vi "FaceDetectionTester.vi"() -> ()   [LabVIEW 2017]
uses:
  Camera_IMAQdx_class/typedefs/Configuration--Cluster.ctl
  Camera_IMAQdx_class/Camera_IMAQdx.lvclass
  ImageFacialDetection_class/ImageFacialDetection.lvclass
  <userlib>/_OpenG.lib/comparison/comparison.llb/Boolean Changed__ogtk.vi
panel:
  in  "Refresh List":bool
  in  "Find Faces":bool
  in  "Connect to Camera":bool
  in  "Cameras":u16(ring) items=["VMware Virtual USB Video Device "]
  out "Image":picture
  in  "OK":bool
  out "Frame Number:":u32
  out "Connected":bool
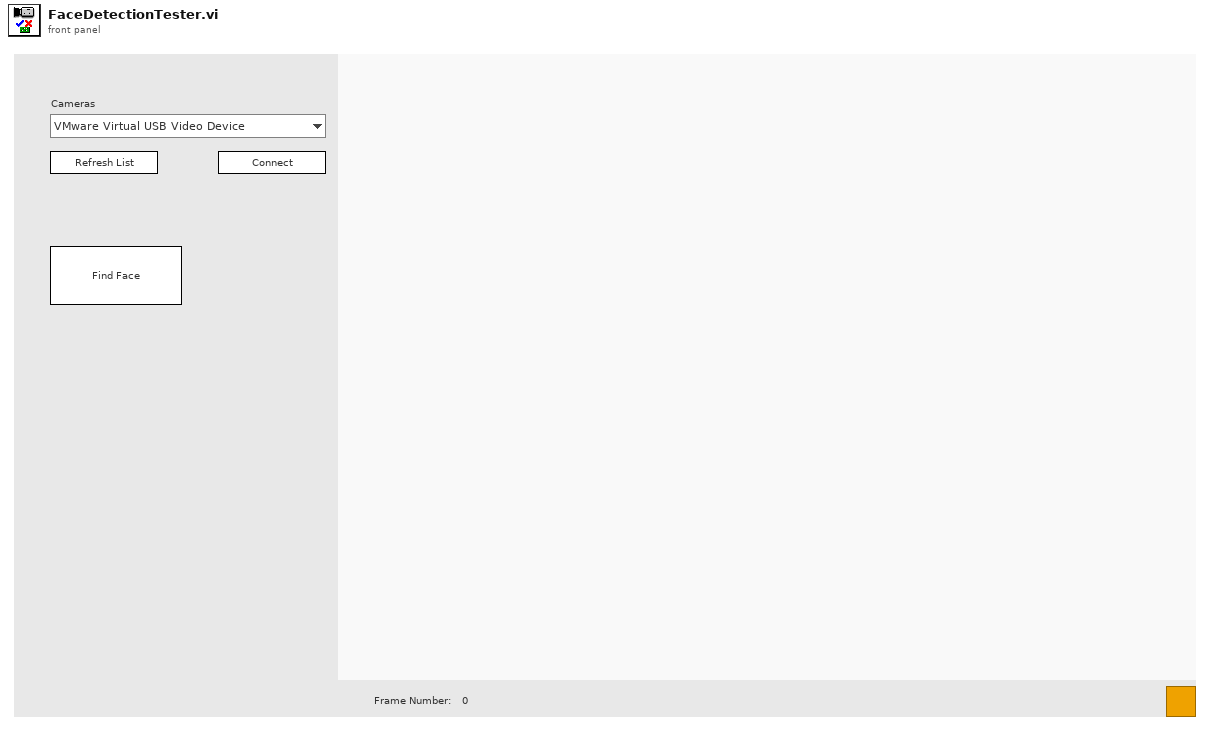
[diagram p1: front panel]
types:
  T1 = typedef "Camera_IMAQdx.lvclass/Configuration--Cluster.ctl" = cluster{"Camera Interface Name":string, "Number of Buffers":u32, "Image Name":string}
  T2 = enum32{"invalid app kind", "Development System", "Run Time System", "Student Edition", "Embedded LabVIEW", "Evaluation", "Custom"}
  T3 = enum8{"Enabled", "Disabled", "Disabled and Grayed Out"}
  T4 = enum32{"Invalid", "Standard", "Closed", "Hidden", "Minimized", "Maximized"}
  T5 = cluster{"Core":cluster{"Current VI Reference":refnum<vi>, "Close Panel on Exit?":bool}, "Camera.IMAQdx":refnum<class "Camera_IMAQdx.lvclass">, "All Camera Interfaces":string[], "Connected":bool, "Grabbing":bool, "ImageFacialDetection":refnum<class "ImageFacialDetection.lvclass">}
  T6 = cluster{"Current VI Reference":refnum<vi>, "Close Panel on Exit?":bool}
  T7 = typedef "IMAQ Image.ctl" = refnum<image>
  T8 = cluster{"Type":u32, "Version":u32, "Flags":u32, "SerialNumberHigh":u32, "SerialNumberLow":u32, "BusType":u32, "InterfaceName":string, "VendorName":string, "ModelName":string, "CameraFileName":string, "CameraAttributeURL":string}[]
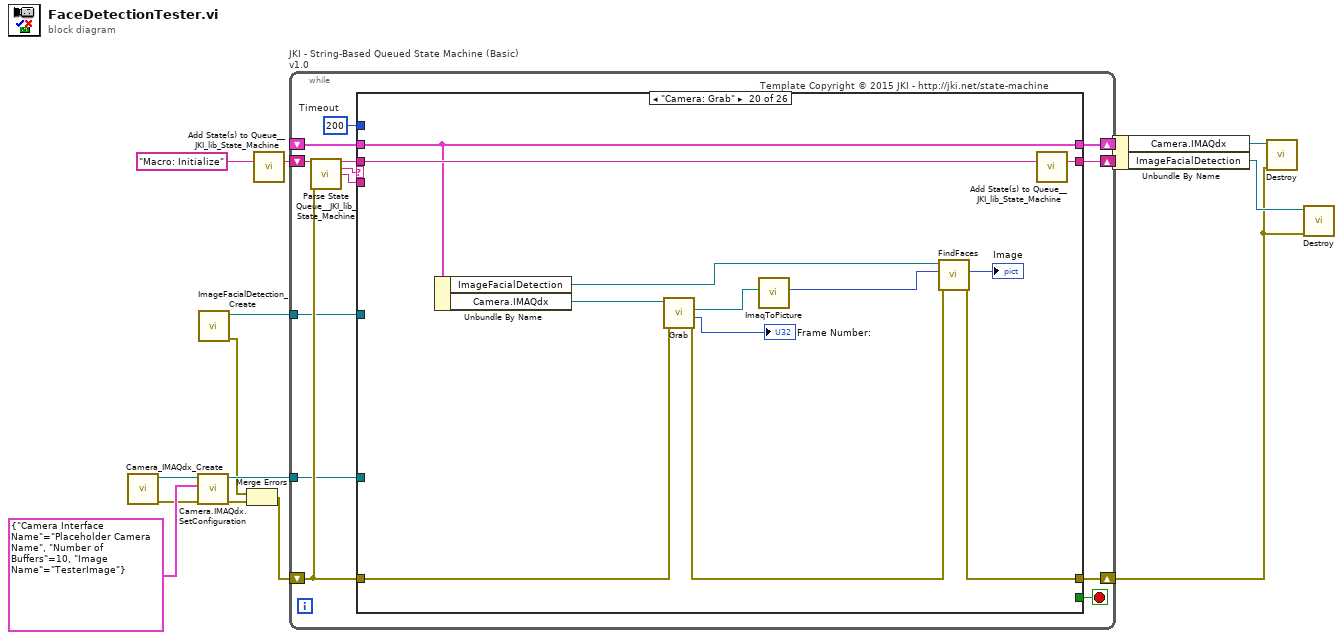
[diagram p0: block diagram]
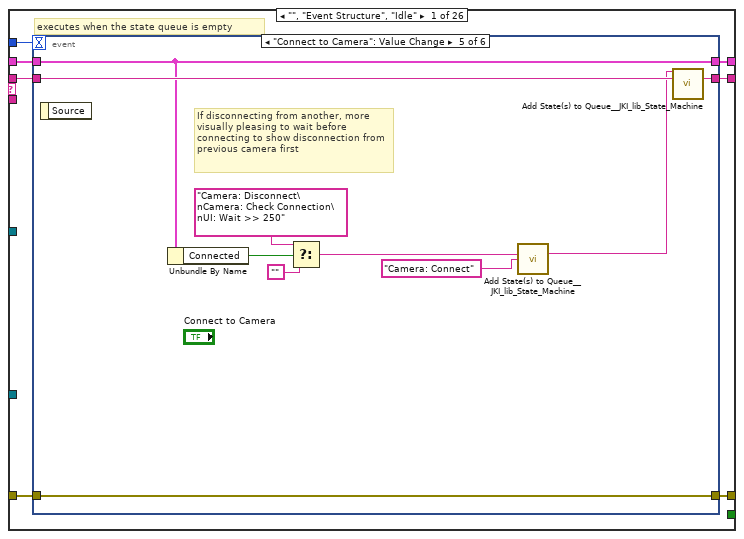
[diagram p2: hidden frame]
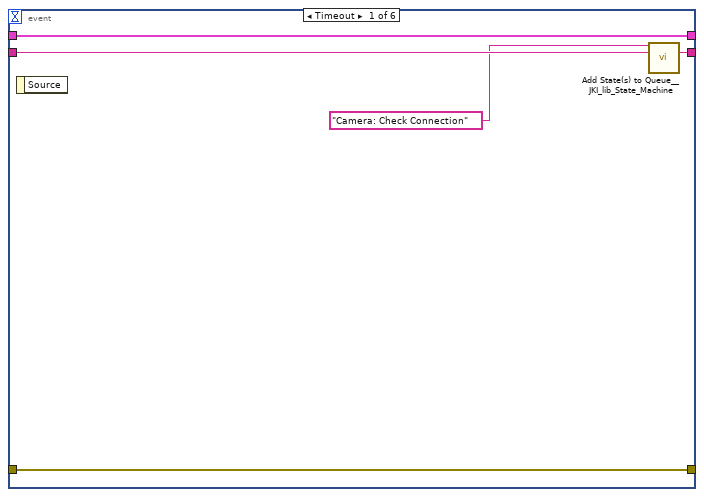
[diagram p3: hidden frame]
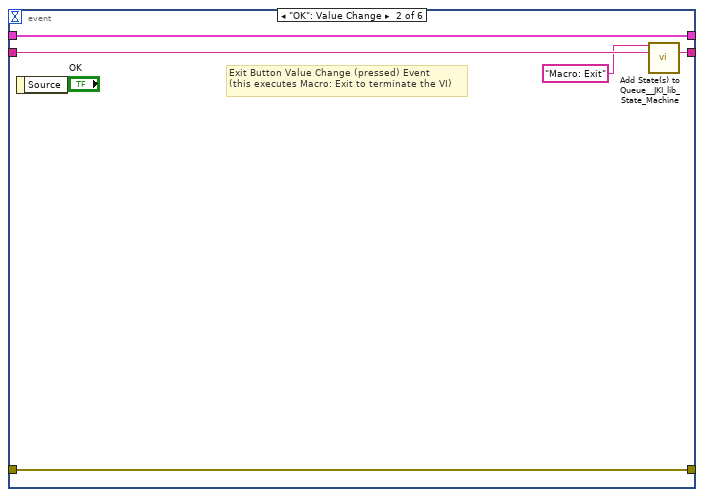
[diagram p4: hidden frame]
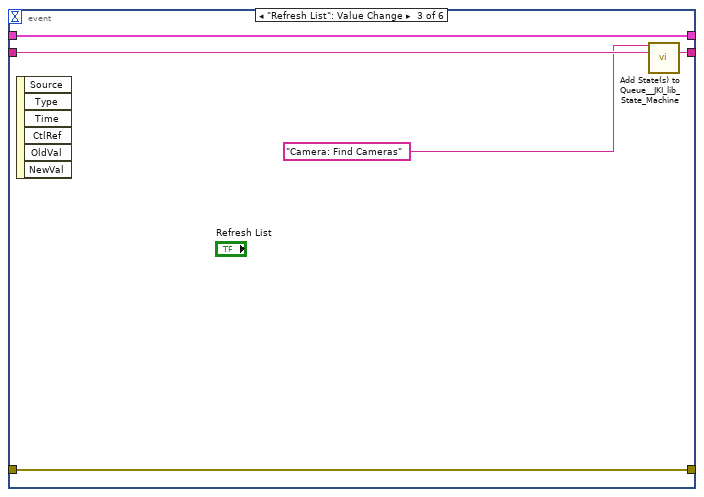
[diagram p5: hidden frame]
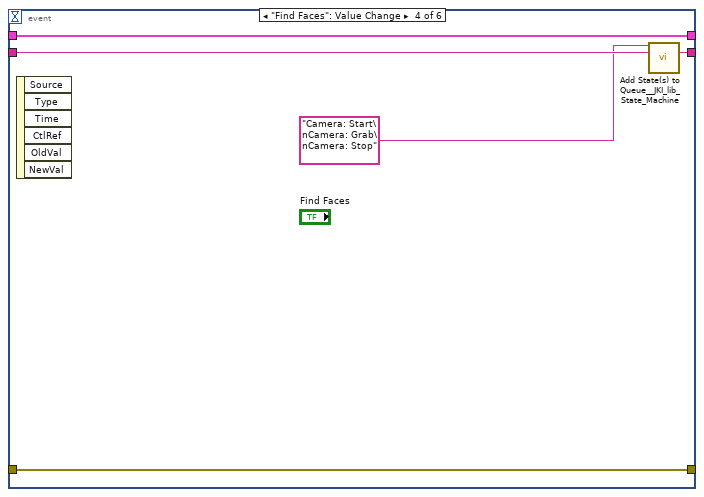
[diagram p6: hidden frame]
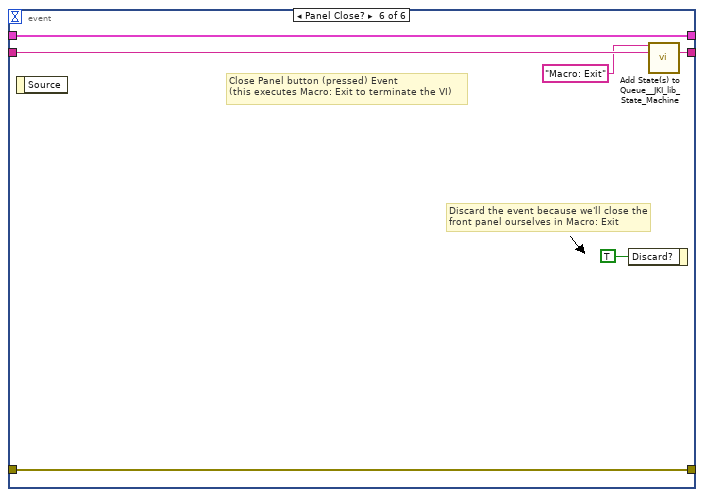
[diagram p7: hidden frame]
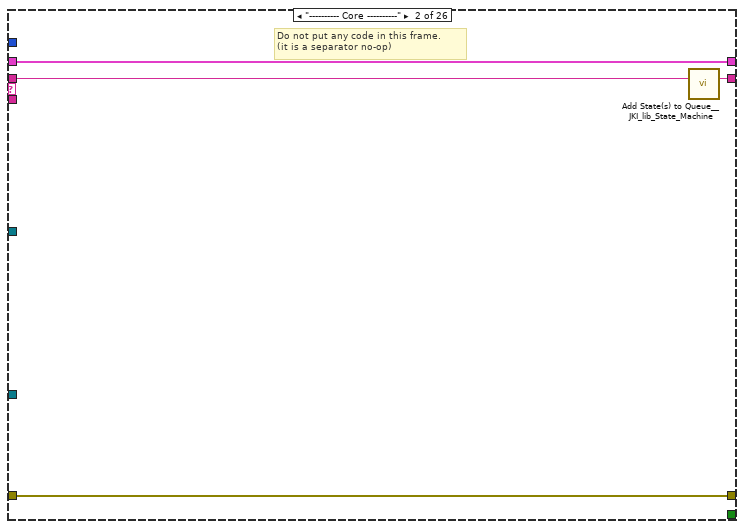
[diagram p8: hidden frame]
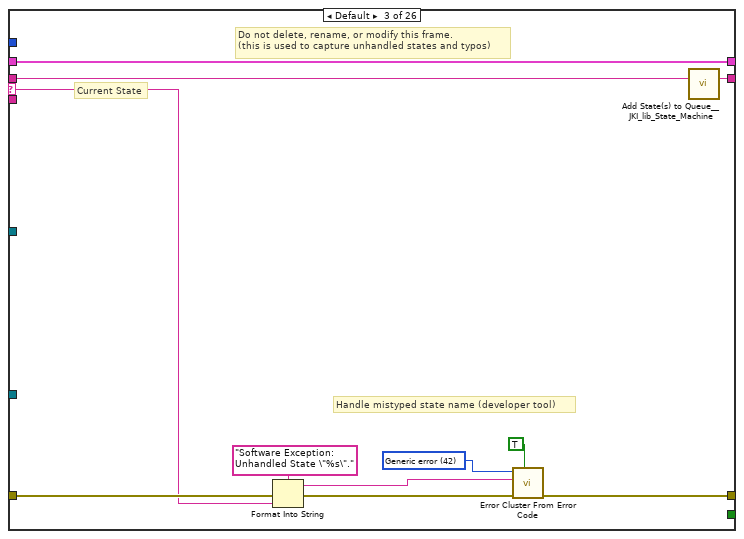
[diagram p9: hidden frame]
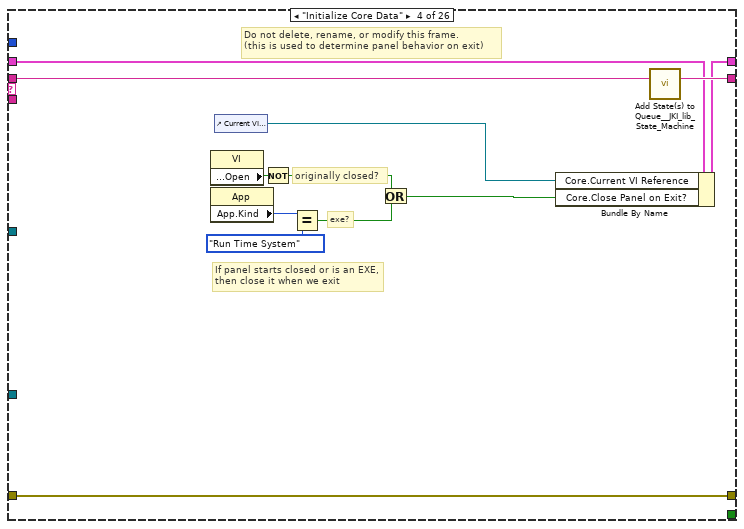
[diagram p10: hidden frame]
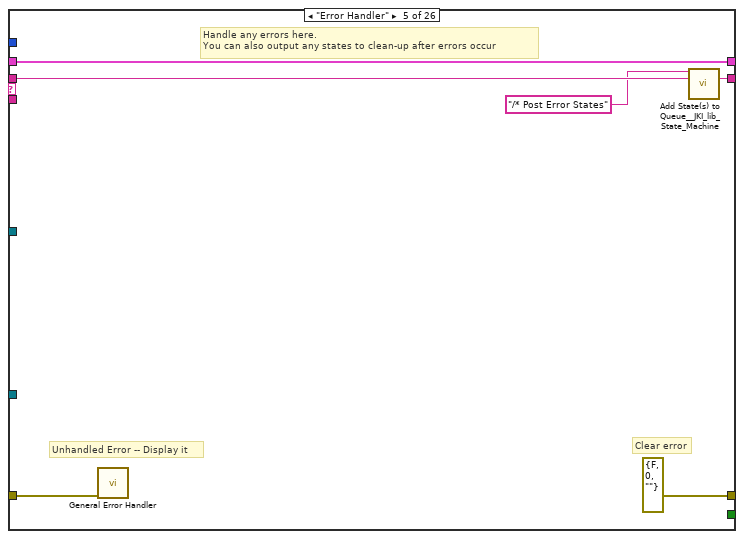
[diagram p11: hidden frame]
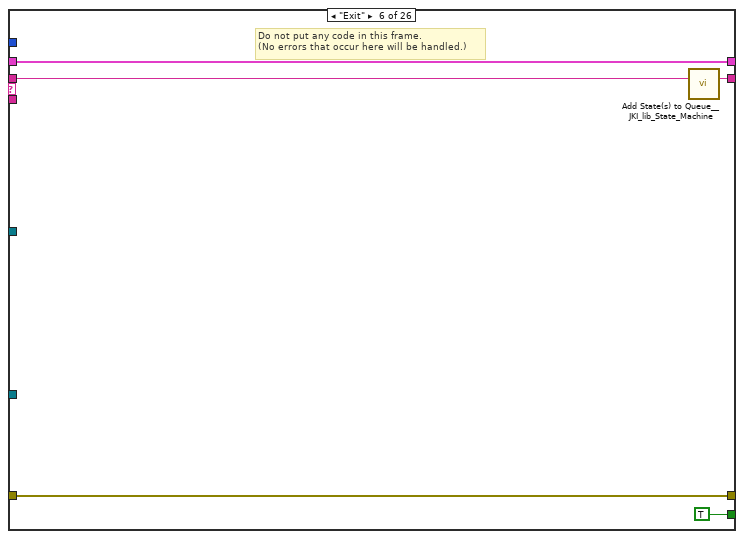
[diagram p12: hidden frame]
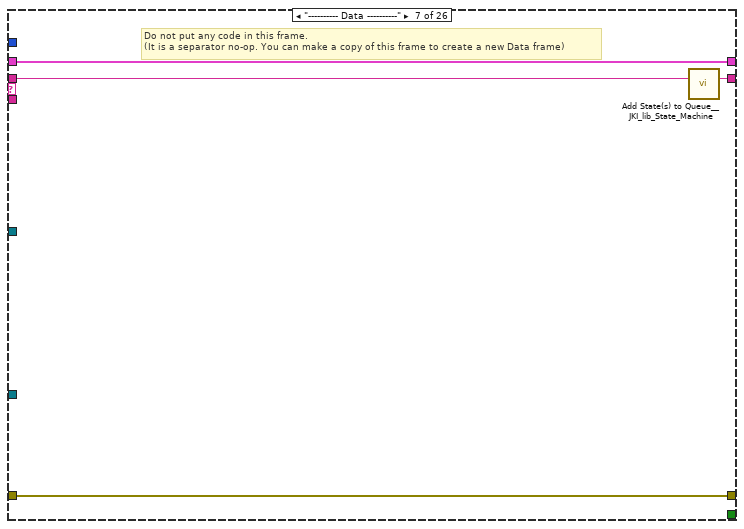
[diagram p13: hidden frame]
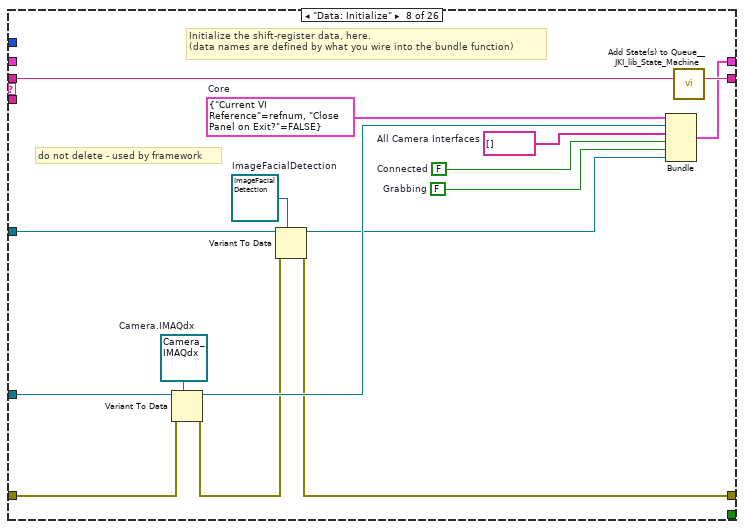
[diagram p14: hidden frame]
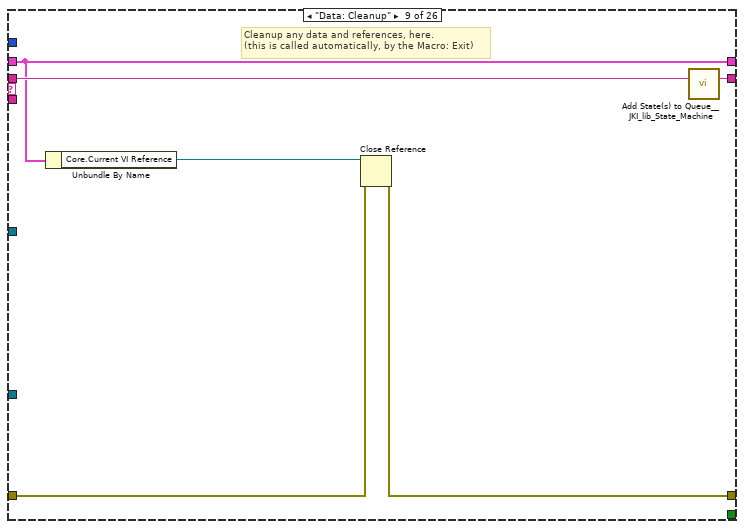
[diagram p15: hidden frame]
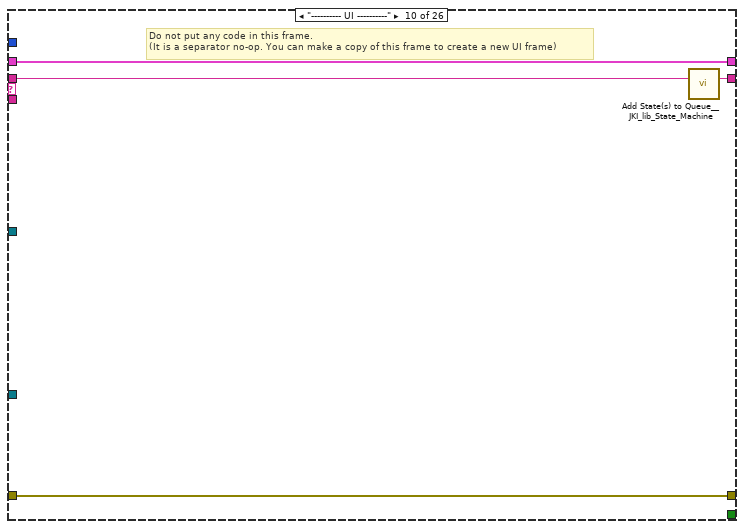
[diagram p16: hidden frame]
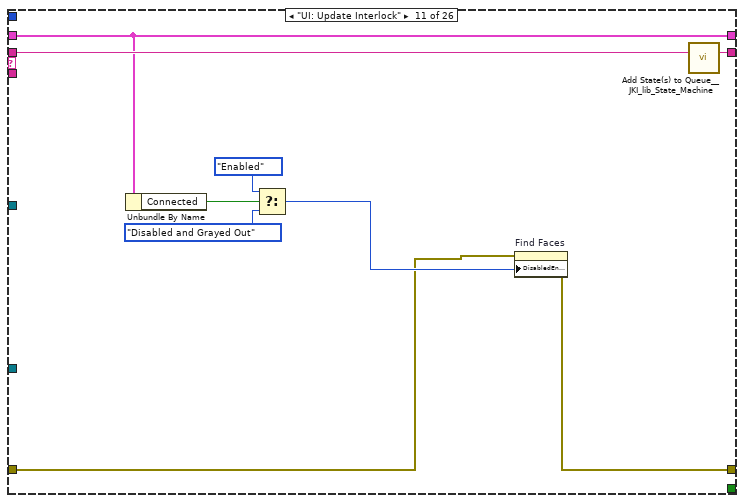
[diagram p17: hidden frame]
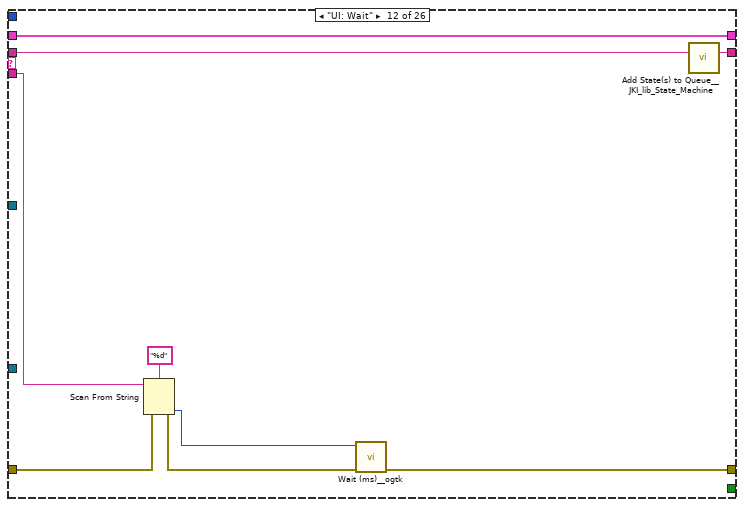
[diagram p18: hidden frame]
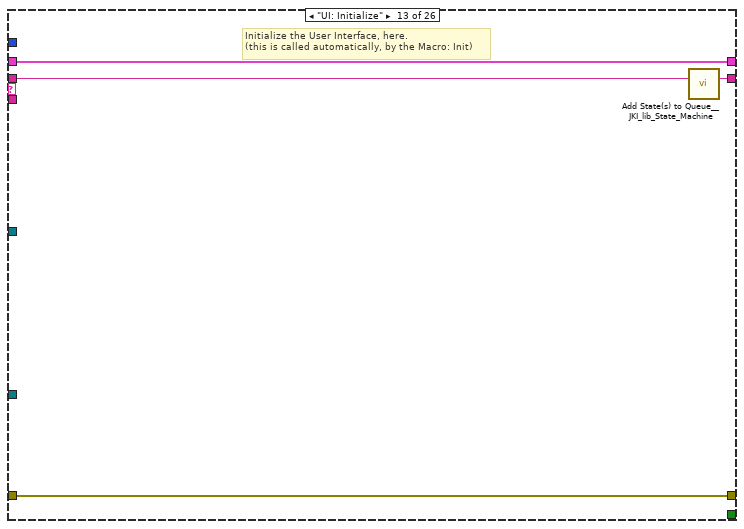
[diagram p19: hidden frame]
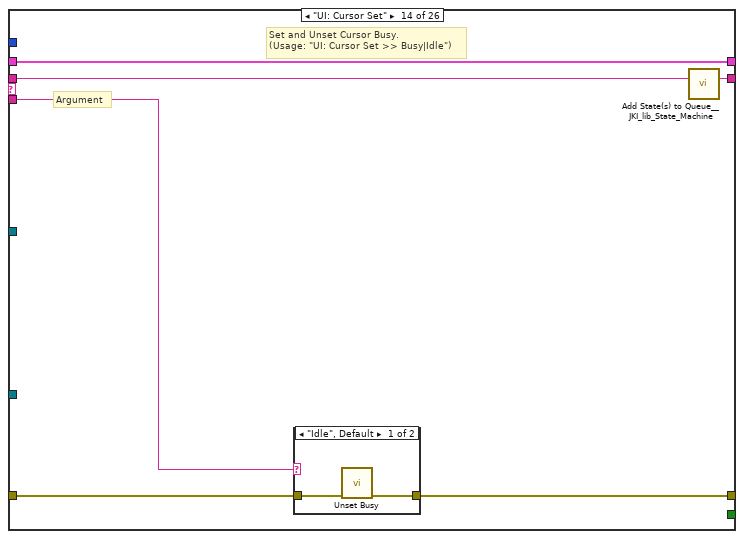
[diagram p20: hidden frame]
diagram:
  n1 = call "Camera_IMAQdx_Create.vi"() -> ("error out"=w7:errorcluster, "reference out"=w12:refnum<class "Camera_IMAQdx.lvclass">)  [unwired: 10 in]
  n2 = call "Camera.IMAQdx.SetConfiguration.vi"("error in (no error)"=w7, "Configuration"=T1 {"Camera Interface Name"="Placeholder Camera Name", "Number of Buffers"=10, "Image Name"="TesterImage"}, "reference in"=w12) -> ("error out"=w6:errorcluster, "reference out"=w9:refnum<class "Camera_IMAQdx.lvclass">)  [unwired: 7 in]
  n3 = call "ImageFacialDetection_Create.vi"() -> ("error out"=w3:errorcluster, "reference out"=w5:refnum<class "ImageFacialDetection.lvclass">)  [unwired: 10 in]
  n4 = Merge Errors(w3, w6) -> (w4:errorcluster)
  n5 = call <vilib>:"Add State(s) to Queue__JKI_lib_State_Machine.vi"("State(s) in (\"\")"="Macro: Initialize") -> ("States Out"=w14:string)  [unwired: 14 in]
  n6 = while "JKI - String-Based Queued State Machine (Basic) v1.0" {
    shift-right: [w20] -> w11
    shift-left: _ -> [w19]
    shift-right: [w23] -> w1
    shift-left: w4 -> [w17]
    shift-right: [w22] -> _
    shift-left: w14 -> [w24]
    tunnel: w9 -> [w16]
    tunnel: w5 -> [w15]
    stop <- w21 stop-if-true
    w18 = 200  # Timeout
    # "Template Copyright © 2015 JKI - http://jki.net/state-machine"
    n7 = call <vilib>:"Parse State Queue__JKI_lib_State_Machine.vi"("State Queue"=w24, "Error In (no error)"=w17) -> ("Remaining States"=w26:string, "Current State"=w27:string, "Arguments"=w25:string)  [unwired: 11 in]
    n8 = case shown="\"Camera: Grab\"" w27 {
      selector: w27 -> [_ _ w75 _ _ _ _ _ _ _ _ _ _ _ _ _ _ _ _ _ _ _ _ _ _ _]
      tunnel: w26 -> [w34 w74 w79 w97 w103 w108 w112 w128 w134 w138 w147 w156 w160 w166 w177 w203 w208 w227 w231 w243 w255 w264 w273 w284 w301 w307]
      tunnel: w25 -> [_ _ _ _ _ _ _ _ _ _ _ w152 _ w161 w171 _ _ _ _ _ _ _ _ _ _ _]
      tunnel: w19 -> [w32 w71 w77 w88 w100 w106 w109 _ w129 w135 w145 w154 w158 w164 w173 w200 w205 w224 w228 w241 w250 w257 w268 w276 w299 w305]
      tunnel: [w31 w72 w81 w94 errorcluster {"status"=FALSE, "code"=0, "source"=""} ("error out") w105 w110 w113 w130 w136 w140 w153 w157 w162 w174 w201 w206 w225 w229 w232 w251 w260 w269 w279 w291 w302] -> w23
      tunnel: w17 -> [w30 w72 w80 w94 w99 w105 w110 w120 w131 w136 w139 w149 w157 w163 w175 w201 w206 w225 w229 w239 w252 w261 w270 w278 w293 w303]
      tunnel: [w33 w73 w78 w96 w102 w107 w111 w127 w133 w137 w146 w155 w159 w165 w176 w202 w207 w226 w230 w242 w254 w263 w272 w283 w300 w306] -> w22
      tunnel: [_ _ _ _ _ TRUE _ _ _ _ _ _ _ _ _ _ _ _ _ _ _ _ _ _ _ _] -> w21
      tunnel: [w29 w71 w77 w95 w100 w106 w109 w126 w129 w135 w145 w154 w158 w164 w173 w200 w205 w224 w228 w241 w249 w256 w267 w275 w299 w305] -> w20
      tunnel: w18 -> [w28 _ _ _ _ _ _ _ _ _ _ _ _ _ _ _ _ _ _ _ _ _ _ _ _ _]
      tunnel: w16 -> [_ _ _ _ _ _ _ w124 _ _ _ _ _ _ _ _ _ _ _ _ _ _ _ _ _ _]
      tunnel: w15 -> [_ _ _ _ _ _ _ w116 _ _ _ _ _ _ _ _ _ _ _ _ _ _ _ _ _ _]
      frame "", "Event Structure", "Idle" {
        # "executes when the state queue is empty"
        n9 = event shown="[4] \"Connect to Camera\": Value Change" {
          selector: _ -> [_ _ _ _ _ _]
          dyn-events: _ -> [_ _ _ _ _ _]
          timeout: w28 -> [_ _ _ _ _ _]
          tunnel: w34 -> [w39 w44 w49 w54 w64 w70]
          tunnel: [w38 w43 w48 w53 w63 w69] -> w33
          tunnel: w32 -> [w36 w41 w46 w51 w61 w67]
          tunnel: [w37 w42 w47 w52 w62 w68] -> w31
          tunnel: w30 -> [w37 w42 w47 w52 w62 w68]
          tunnel: [w36 w41 w46 w51 w61 w67] -> w29
          event Timeout {
            n10 = event-data() -> ()  [unwired: 1 in, 1 out]
            n11 = call <vilib>:"Add State(s) to Queue__JKI_lib_State_Machine.vi"("State(s) in Front (\"\")"="Camera: Check Connection", "State(s) in (\"\")"=w39) -> ("States Out"=w38:string)  [unwired: 13 in]
          }
          event "OK": Value Change {
            # "Exit Button Value Change (pressed) Event\n(this executes Macro: Exit to terminate the VI)"
            n12 = event-data() -> ()  [unwired: 1 in, 1 out]
            n13 = call <vilib>:"Add State(s) to Queue__JKI_lib_State_Machine.vi"("State(s) in Front (\"\")"="Macro: Exit", "State(s) in (\"\")"=w44) -> ("States Out"=w43:string)  [unwired: 13 in]
          }
          event "Refresh List": Value Change {
            n14 = event-data() -> ()  [unwired: 1 in, 6 out]
            n15 = call <vilib>:"Add State(s) to Queue__JKI_lib_State_Machine.vi"("State(s) in Front (\"\")"="Camera: Find Cameras", "State(s) in (\"\")"=w49) -> ("States Out"=w48:string)  [unwired: 13 in]
          }
          event "Find Faces": Value Change {
            n16 = event-data() -> ()  [unwired: 1 in, 6 out]
            n17 = call <vilib>:"Add State(s) to Queue__JKI_lib_State_Machine.vi"("State(s) in Front (\"\")"="Camera: Start\nCamera: Grab\nCamera: Stop", "State(s) in (\"\")"=w54) -> ("States Out"=w53:string)  [unwired: 13 in]
          }
          event "Connect to Camera": Value Change {
            # "If disconnecting from another, more visually pleasing to wait before connecting to show disconnection from previous camera first"
            n18 = event-data() -> ()  [unwired: 1 in, 1 out]
            n19 = Unbundle By Name(w61) -> ("Connected"=w60:bool)
            n20 = Select(t="Camera: Disconnect\nCamera: Check Connection\nUI: Wait >> 250", s=w60, f="") -> (s? t:f=w57:string)
            n21 = call <vilib>:"Add State(s) to Queue__JKI_lib_State_Machine.vi"("State(s) in (\"\")"=w57, "State(s) at Back (\"\")"="Camera: Connect") -> ("States Out"=w55:string)  [unwired: 13 in]
            n22 = call <vilib>:"Add State(s) to Queue__JKI_lib_State_Machine.vi"("State(s) in Front (\"\")"=w55, "State(s) in (\"\")"=w64) -> ("States Out"=w63:string)  [unwired: 13 in]
          }
          event Panel Close? {
            # "Discard the event because we'll close the front panel ourselves in Macro: Exit"
            # "Close Panel button (pressed) Event\n(this executes Macro: Exit to terminate the VI)"
            n23 = event-data() -> ()  [unwired: 1 in, 1 out]
            n24 = event-data("Discard?"=TRUE) -> ()  [unwired: 1 in, 1 out]
            n25 = call <vilib>:"Add State(s) to Queue__JKI_lib_State_Machine.vi"("State(s) in Front (\"\")"="Macro: Exit", "State(s) in (\"\")"=w70) -> ("States Out"=w69:string)  [unwired: 13 in]
          }
        }
      }
      frame "---------- Core ----------" {
        # "Do not put any code in this frame.\n(it is a separator no-op)"
        n26 = call <vilib>:"Add State(s) to Queue__JKI_lib_State_Machine.vi"("State(s) in (\"\")"=w74) -> ("States Out"=w73:string)  [unwired: 14 in]
      }
      frame Default {
        w84 = 42 items=["No error", "Argument error", "Memory is full", "Out of zone", "End of file", "File already open", "Generic file I/O error", "File not found", "File permission error", "Disk is full", "Duplicate path", "Too many files open", "System feature not enabled", "Resource file not found", "Cannot add resource", "Resource not found", "Image not found", "Image memory error", "Pen does not exist", "Config type invalid", "Config token not found", "Config parse error", "Config memory error", "Bad external code format", "Bad external code offset", "External code not present", "Null window", "Destroy window error", "Null menu", "Print aborted", "Bad print record", "Print driver error", "Windows error during printing", "Memory error during printing", "Print dialog error", "Generic print error", "Invalid device refnum", "Device not found", "Device parameter error", "Device unit error", "Cannot open device", "Device call aborted", "Generic error", "Cancelled by user", "Object ID too low", "Object ID too high", "Object not in heap", "Unknown heap", "Unknown object (invalid DefProc)", "Unknown object (DefProc not in table)", "Message out of range", "Invalid (null) method", "Unknown message", "Manager call not supported", "Bad address", "Network operation in progress", "Network operation timed out", "Connection is busy", "Network attribute not supported", "Network error", "Address in use", "System out of memory", "Connection aborted", "Connection refused", "Not connected", "Already connected", "Connection closed", "Initialization error (interapplication manager)", "Bad occurrence", "Wait on unbound occurrence handler", "Occurrence queue overflow", "Datalog type conflict", "Unused", "Unrecognized type (interapplication manager)", "Memory corrupt", "Failed to make temporary DLL", "Old CIN version", "Drag socket not found", "Failed to load drop-object", "Failed to register OLE object", "Failed to release OLE object", "Format specifier type mismatch", "Unknown format specifier", "Too few format specifiers", "Too many format specifiers", "Scan failed", "Newer CIN version", "Error converting to variant", "Runtime menu error", "Password tampered", "Variant attribute not found", "Incompatible variant data type", "Event data is not available", "Event Store is not present", "Occurrence is not found", "Event Queue is not created", "Event info is not available", "Refnum passed is NULL", "Error retrieving Class GUID", "Error retrieving CoClass GUID", "Error retrieving TypeLib GUID.", "Bad built application magic bytes.", "Specific driver is different from the specific driver associated with the Logical Name.", "There is no session opened to the class driver.", "Max Error", "MAX - Error with config objects", "MAX - Error loading configuration", "MAX - Group not supported"]
        # "Current State"
        # "Do not delete, rename, or modify this frame.\n(this is used to capture unhandled states and typos)"
        # "Handle mistyped state name (developer tool)"
        n27 = Format Into String(format string="Software Exception: Unhandled State \"%s\"." ("message"), error in=w80, w75) -> (resulting string=w83:string, error out=w82:errorcluster)  [unwired: 1 in]
        n28 = call <vilib>:"Error Cluster From Error Code.vi"("show call chain? (False)"=TRUE, "error in (no error)"=w82, "error message (\"\")"=w83, "error code (0)"=w84) -> ("error out"=w81:errorcluster)  [unwired: 5 in]
        n29 = call <vilib>:"Add State(s) to Queue__JKI_lib_State_Machine.vi"("State(s) in (\"\")"=w79) -> ("States Out"=w78:string)  [unwired: 14 in]
      }
      frame "Initialize Core Data" {
        # "Do not delete, rename, or modify this frame.\n(this is used to determine panel behavior on exit)"
        # "originally closed?"
        # "exe?"
        # "If panel starts closed or is an EXE, then close it when we exit"
        n30 = property class="VI"() -> ("Front Panel.Open"=w93:bool)  [unwired: 2 in, 2 out]
        n31 = property class="App"() -> ("App.Kind"=w92:T2)  [unwired: 2 in, 2 out]
        n32 = control-ref of="Current VI Reference"() -> (w86:refnum<vi>)
        n33 = Not(x=w93) -> (.not. x?=w90:bool)
        n34 = Equal?(x=w92, y=T2."Run Time System" ("Application:Kind")) -> (x = y?=w89:bool)
        n35 = Or(x=w90, y=w89) -> (x .or. y?=w87:bool)
        n36 = Bundle By Name(cluster=w88, "Core.Current VI Reference"=w86, "Core.Close Panel on Exit?"=w87) -> (w95:T5)
        n37 = call <vilib>:"Add State(s) to Queue__JKI_lib_State_Machine.vi"("State(s) in (\"\")"=w97) -> ("States Out"=w96:string)  [unwired: 14 in]
      }
      frame "Error Handler" {
        # "Unhandled Error -- Display it"
        # "Handle any errors here.\nYou can also output any states to clean-up after errors occur"
        # "Clear error"
        n38 = call <vilib>:"General Error Handler.vi"("error in (no error)"=w99) -> ()  [unwired: 10 in, 5 out]
        n39 = call <vilib>:"Add State(s) to Queue__JKI_lib_State_Machine.vi"("State(s) in Front (\"\")"="/* Post Error States", "State(s) in (\"\")"=w103) -> ("States Out"=w102:string)  [unwired: 13 in]
      }
      frame "Exit" {
        # "Do not put any code in this frame.\n(No errors that occur here will be handled.)"
        n40 = call <vilib>:"Add State(s) to Queue__JKI_lib_State_Machine.vi"("State(s) in (\"\")"=w108) -> ("States Out"=w107:string)  [unwired: 14 in]
      }
      frame "---------- Data ----------" {
        # "Do not put any code in this frame.\n(It is a separator no-op. You can make a copy of this frame to create a new Data frame)"
        n41 = call <vilib>:"Add State(s) to Queue__JKI_lib_State_Machine.vi"("State(s) in (\"\")"=w112) -> ("States Out"=w111:string)  [unwired: 14 in]
      }
      frame "Data: Initialize" {
        w117 = refnum<class "ImageFacialDetection.lvclass"> refnum  # ImageFacialDetection
        w118 = FALSE  # Grabbing
        w119 = FALSE  # Connected
        w122 = refnum<class "Camera_IMAQdx.lvclass"> refnum  # Camera.IMAQdx
        w123 = string[] []  # All Camera Interfaces
        w125 = T6 {"Current VI Reference"=refnum, "Close Panel on Exit?"=FALSE}  # Core
        # "do not delete - used by framework"
        # "Initialize the shift-register data, here.\n(data names are defined by what you wire into the bundle function)"
        n42 = Variant To Data(error in=w120, type=w122, Variant=w124) -> (data=w121:refnum<class "Camera_IMAQdx.lvclass">, error out=w114:errorcluster)
        n43 = Variant To Data(error in=w114, type=w117, Variant=w116) -> (data=w115:refnum<class "ImageFacialDetection.lvclass">, error out=w113:errorcluster)
        n44 = Bundle("Core"=w125, "Camera.IMAQdx"=w121, "All Camera Interfaces"=w123, "Connected"=w119, "Grabbing"=w118, "ImageFacialDetection"=w115) -> (w126:T5)  [unwired: 1 in]
        n45 = call <vilib>:"Add State(s) to Queue__JKI_lib_State_Machine.vi"("State(s) in (\"\")"=w128) -> ("States Out"=w127:string)  [unwired: 14 in]
      }
      frame "Data: Cleanup" {
        # "Cleanup any data and references, here.\n(this is called automatically, by the Macro: Exit)"
        n46 = Unbundle By Name(w129) -> ("Core.Current VI Reference"=w132:refnum<vi>)
        n47 = Close Reference(reference=w132, error in (no error)=w131) -> (error out=w130:errorcluster)
        n48 = call <vilib>:"Add State(s) to Queue__JKI_lib_State_Machine.vi"("State(s) in (\"\")"=w134) -> ("States Out"=w133:string)  [unwired: 14 in]
      }
      frame "---------- UI ----------" {
        # "Do not put any code in this frame.\n(It is a separator no-op. You can make a copy of this frame to create a new UI frame)"
        n49 = call <vilib>:"Add State(s) to Queue__JKI_lib_State_Machine.vi"("State(s) in (\"\")"=w138) -> ("States Out"=w137:string)  [unwired: 14 in]
      }
      frame "UI: Update Interlock" {
        n50 = Unbundle By Name(w145) -> ("Connected"=w144:bool)
        n51 = Select(t=T3."Enabled" ("Disabled"), s=w144, f=T3."Disabled and Grayed Out" ("Disabled")) -> (s? t:f=w141:T3)
        n52 = property on="Find Faces" class="Bool"(error in=w139, "DisabledEnum"=w141) -> (error out=w140:errorcluster)  [unwired: 1 in, 1 out]
        n53 = call <vilib>:"Add State(s) to Queue__JKI_lib_State_Machine.vi"("State(s) in (\"\")"=w147) -> ("States Out"=w146:string)  [unwired: 14 in]
      }
      frame "UI: Wait" {
        n54 = Scan From String(format string="%d", input string=w152, error in=w149) -> (error out=w148:errorcluster, output 1=w150:i32)  [unwired: 2 in, 2 out]
        n55 = call <userlib>:"Wait (ms)__ogtk.vi"("error in (no error)"=w148, "milliseconds to wait"=w150) -> ("error out"=w153:errorcluster)  [unwired: 8 in, 1 out]
        n56 = call <vilib>:"Add State(s) to Queue__JKI_lib_State_Machine.vi"("State(s) in (\"\")"=w156) -> ("States Out"=w155:string)  [unwired: 14 in]
      }
      frame "UI: Initialize" {
        # "Initialize the User Interface, here.\n(this is called automatically, by the Macro: Init)"
        n57 = call <vilib>:"Add State(s) to Queue__JKI_lib_State_Machine.vi"("State(s) in (\"\")"=w160) -> ("States Out"=w159:string)  [unwired: 14 in]
      }
      frame "UI: Cursor Set" {
        # "Argument"
        # "Set and Unset Cursor Busy.\n(Usage: \"UI: Cursor Set >> Busy|Idle\")"
        n58 = case shown="\"Idle\", Default" w161 {
          tunnel: w163 -> [w168 w170]
          tunnel: [w167 w169] -> w162
          frame "Idle", Default {
            n59 = call <vilib>:"Unset Busy.vi"("error in (no error)"=w168) -> ("error out"=w167:errorcluster)  [unwired: 10 in]
          }
          frame "Busy" {
            n60 = call <vilib>:"Set Busy.vi"("error in (no error)"=w170) -> ("error out"=w169:errorcluster)  [unwired: 9 in, 1 out]
          }
        }
        n61 = call <vilib>:"Add State(s) to Queue__JKI_lib_State_Machine.vi"("State(s) in (\"\")"=w166) -> ("States Out"=w165:string)  [unwired: 14 in]
      }
      frame "UI: Front Panel State" {
        # "Argument"
        # "Set Front Panel Open or Closed\n(Usage: \"UI: Front Panel State >> Open|Close\")"
        n62 = Unbundle By Name(w173) -> ("Core.Current VI Reference"=w172:refnum<vi>)
        n63 = case shown="\"Open\", Default" w171 {
          tunnel: w175 -> [w181 w194]
          tunnel: [w183 w195] -> w174
          tunnel: w172 -> [w182 w192]
          frame "Open", Default {
            n64 = property class="VI"(reference=w182, error in=w181) -> (reference out=w179:refnum<vi>, error out=w180:errorcluster, "Front Panel.Open"=w178:bool)
            n65 = case shown="False" w178 {
              tunnel: [w186 w189] -> w183
              tunnel: w180 -> [w185 w189]
              tunnel: w179 -> [w184 _]
              frame False {
                n66 = invoke class="VI" method="FP.Open"(reference=w184, error in=w185, "Activate"=TRUE, "State"=T4."Standard") -> (error out=w186:errorcluster)  [unwired: 1 in, 4 out]
              }
              frame True {
              }
            }
          }
          frame "Close" {
            n67 = property class="VI"(reference=w192, error in=w194) -> (reference out=w191:refnum<vi>, error out=w193:errorcluster, "Front Panel.Open"=w190:bool)
            n68 = case shown="True" w190 {
              tunnel: [w196 w199] -> w195
              tunnel: w193 -> [w196 w198]
              tunnel: w191 -> [_ w197]
              frame False {
              }
              frame True {
                n69 = invoke class="VI" method="FP.Close"(reference=w197, error in=w198) -> (error out=w199:errorcluster)  [unwired: 1 in, 2 out]
              }
            }
          }
        }
        n70 = call <vilib>:"Add State(s) to Queue__JKI_lib_State_Machine.vi"("State(s) in (\"\")"=w177) -> ("States Out"=w176:string)  [unwired: 14 in]
      }
      frame "---------- Macro ----------" {
        # "Do not put any code in this frame.\n(It is a separator no-op. You can make a copy of this frame to create a new Macro frame)"
        n71 = call <vilib>:"Add State(s) to Queue__JKI_lib_State_Machine.vi"("State(s) in (\"\")"=w203) -> ("States Out"=w202:string)  [unwired: 14 in]
      }
      frame "Macro: Initialize" {
        w204 = "Data: Initialize\nInitialize Core Data\nUI: Initialize\nCamera: Find Cameras\nUI: Update Interlock\nUI: Front Panel State >> Open"  # Data: Initialize Initialize Core Data UI: Initialize Camera: Find Cameras UI: Update Interlock UI: Front Panel State >> Open
        # "Initialization Macro\n(This is called once, when the VI starts)"
        n72 = call <vilib>:"Add State(s) to Queue__JKI_lib_State_Machine.vi"("State(s) in Front (\"\")"=w204, "State(s) in (\"\")"=w208) -> ("States Out"=w207:string)  [unwired: 13 in]
      }
      frame "Macro: Exit" {
        # "Exit Macro\n(This is called once, when the VI exits)"
        n73 = Unbundle By Name(w224) -> ("Grabbing"=w213:bool, "Connected"=w212:bool, "Core.Close Panel on Exit?"=w223:bool)
        n74 = Select(t="Camera: Stop", s=w213, f="") -> (s? t:f=w211:string)
        n75 = Select(t="Camera: Disconnect", s=w212, f="") -> (s? t:f=w210:string)
        n76 = Select(t="UI: Front Panel State >> Close", s=w223, f="") -> (s? t:f=w220:string)
        n77 = call <vilib>:"Add State(s) to Queue__JKI_lib_State_Machine.vi"("State(s) in Front (\"\")"=w211, "State(s) in (\"\")"=w210) -> ("States Out"=w209:string)  [unwired: 13 in]
        n78 = call <vilib>:"Add State(s) to Queue__JKI_lib_State_Machine.vi"("State(s) in Front (\"\")"=w209, "State(s) in (\"\")"=w220, "State(s) at Back (\"\")"="Data: Cleanup\nExit") -> ("States Out"=w218:string)  [unwired: 12 in]
        n79 = call <vilib>:"Add State(s) to Queue__JKI_lib_State_Machine.vi"("State(s) in Front (\"\")"=w218, "State(s) in (\"\")"=w227) -> ("States Out"=w226:string)  [unwired: 13 in]
      }
      frame "---------- Camera ----------" {
        # "Template Separator\n(You can make a copy of, or modify, this frame)"
        n80 = call <vilib>:"Add State(s) to Queue__JKI_lib_State_Machine.vi"("State(s) in (\"\")"=w231) -> ("States Out"=w230:string)  [unwired: 14 in]
      }
      frame "Camera: Grab" {
        n81 = Unbundle By Name(w241) -> ("ImageFacialDetection"=w236:refnum<class "ImageFacialDetection.lvclass">, "Camera.IMAQdx"=w240:refnum<class "Camera_IMAQdx.lvclass">)
        n82 = call-dynamic "Grab.vi"("error in (no error)"=w239, "reference in"=w240) -> ("error out"=w233:errorcluster, "Frame Number"=→"Frame Number:":u32, "Image Out"=w237:T7)  [unwired: 6 in, 1 out]
        n83 = call "ImaqToPicture.vi"("Image"=w237) -> ("Picture"=w235:picture)  [unwired: 10 in]
        n84 = call "FindFaces.vi"("error in (no error)"=w233, "image"=w235, "reference in"=w236) -> ("error out"=w232:errorcluster, "image with faces"=→"Image":picture)  [unwired: 6 in, 1 out]
        n85 = call <vilib>:"Add State(s) to Queue__JKI_lib_State_Machine.vi"("State(s) in (\"\")"=w243) -> ("States Out"=w242:string)  [unwired: 14 in]
      }
      frame "Camera: Check Connection" {
        n86 = Unbundle By Name(w250) -> ("Camera.IMAQdx"=w253:refnum<class "Camera_IMAQdx.lvclass">)
        n87 = call-dynamic "GetConnected.vi"("error in (no error)"=w252, "reference in"=w253) -> ("error out"=w251:errorcluster, "Connected"=w248:bool)  [unwired: 7 in, 1 out]
        "Connected" <- w248
        n88 = call-poly <userlib>:"Data Changed__ogtk.vi"("Boolean"=w248) -> ("Changed"=w247:bool)
        n89 = Bundle By Name(cluster=w250, "Connected"=w248) -> (w249:T5)
        n90 = Select(t="UI: Update Interlock", s=w247, f="") -> (s? t:f=w244:string)
        n91 = call <vilib>:"Add State(s) to Queue__JKI_lib_State_Machine.vi"("State(s) in Front (\"\")"=w244, "State(s) in (\"\")"=w255) -> ("States Out"=w254:string)  [unwired: 13 in]
      }
      frame "Camera: Start" {
        n92 = Unbundle By Name(w257) -> ("Camera.IMAQdx"=w262:refnum<class "Camera_IMAQdx.lvclass">)
        n93 = call-dynamic "StartAcquisition.vi"("error in (no error)"=w261, "reference in"=w262) -> ("error out"=w260:errorcluster)  [unwired: 8 in, 1 out]
        n94 = Unbundle By Name(w260) -> ("status"=w259:bool)
        n95 = Not(x=w259) -> (.not. x?=w258:bool)
        n96 = Bundle By Name(cluster=w257, "Grabbing"=w258) -> (w256:T5)
        n97 = call <vilib>:"Add State(s) to Queue__JKI_lib_State_Machine.vi"("State(s) in (\"\")"=w264) -> ("States Out"=w263:string)  [unwired: 14 in]
      }
      frame "Camera: Stop" {
        n98 = Unbundle By Name(w268) -> ("Camera.IMAQdx"=w271:refnum<class "Camera_IMAQdx.lvclass">)
        n99 = call-dynamic "StopAcquisition.vi"("error in (no error)"=w270, "reference in"=w271) -> ("error out"=w269:errorcluster)  [unwired: 8 in, 1 out]
        n100 = local write "Frame Number:"(u32 0 ("Frame Number:")) -> ()
        n101 = Bundle By Name(cluster=w268, "Grabbing"=FALSE) -> (w267:T5)
        n102 = call <vilib>:"Add State(s) to Queue__JKI_lib_State_Machine.vi"("State(s) in (\"\")"=w273) -> ("States Out"=w272:string)  [unwired: 14 in]
      }
      frame "Camera: Find Cameras" {
        n103 = Unbundle By Name(w276) -> ("Camera.IMAQdx"=w282:refnum<class "Camera_IMAQdx.lvclass">)
        n104 = call "FindCameras.vi"("error in (no error)"=w278, "reference in"=w282) -> ("error out"=w277:errorcluster, "Camera Information Array"=w281:T8)  [unwired: 7 in, 1 out]
        n105 = for {
          tunnel: w281 -> [w290] mode=indexing
          tunnel: [w286] -> w280 mode=indexing
          tunnel: [w285] -> w274 mode=indexing
          n106 = Unbundle By Name(w290) -> ("InterfaceName"=w285:string, "VendorName"=w289:string, "ModelName"=w287:string)
          n107 = call <vilib>:"Space Constant.vi"() -> ("String"=w288:string)
          n108 = Concatenate Strings(w289, w288, w287) -> (w286:string)
        }
        n109 = Bundle By Name(cluster=w276, "All Camera Interfaces"=w274) -> (w275:T5)
        n110 = property on="Cameras" class="Ring (strict)"(error in=w277, "Strings []"=w280) -> (error out=w279:errorcluster)  [unwired: 1 in, 1 out]
        n111 = call <vilib>:"Add State(s) to Queue__JKI_lib_State_Machine.vi"("State(s) in (\"\")"=w284) -> ("States Out"=w283:string)  [unwired: 14 in]
      }
      frame "Camera: Connect" {
        n112 = Unbundle By Name(w299) -> ("Camera.IMAQdx"=w298:refnum<class "Camera_IMAQdx.lvclass">, "All Camera Interfaces"=w296:string[])
        n113 = Index Array(array=w296, index="Cameras") -> (element=w294:string)
        n114 = call "SetCameraInterfaceName.vi"("error in (no error)"=w293, "Camera Interface Name"=w294, "reference in"=w298) -> ("error out"=w292:errorcluster, "reference out"=w297:refnum<class "Camera_IMAQdx.lvclass">)  [unwired: 7 in]
        n115 = call-dynamic "Connect.vi"("error in (no error)"=w292, "reference in"=w297) -> ("error out"=w291:errorcluster)  [unwired: 8 in, 1 out]
        n116 = call <vilib>:"Add State(s) to Queue__JKI_lib_State_Machine.vi"("State(s) in (\"\")"=w301) -> ("States Out"=w300:string)  [unwired: 14 in]
      }
      frame "Camera: Disconnect" {
        n117 = Unbundle By Name(w305) -> ("Camera.IMAQdx"=w304:refnum<class "Camera_IMAQdx.lvclass">)
        n118 = call-dynamic "Disconnect.vi"("error in (no error)"=w303, "reference in"=w304) -> ("error out"=w302:errorcluster)  [unwired: 8 in, 1 out]
        n119 = call <vilib>:"Add State(s) to Queue__JKI_lib_State_Machine.vi"("State(s) in (\"\")"=w307) -> ("States Out"=w306:string)  [unwired: 14 in]
      }
    }
  }
  n120 = Unbundle By Name(w11) -> ("Camera.IMAQdx"=w10:refnum<class "Camera_IMAQdx.lvclass">, "ImageFacialDetection"=w2:refnum<class "ImageFacialDetection.lvclass">)
  n121 = call-dynamic "Destroy.vi"("error in (no error)"=w1, "reference in"=w10) -> ()  [unwired: 8 in, 2 out]
  n122 = call-dynamic "Destroy.vi"("error in (no error)"=w1, "reference in"=w2) -> ()  [unwired: 8 in, 2 out]
